vi "initialise.vi"(8 "error in (no error)":errorcluster, 11 "DL090202FPGAClock in":refnum<class "ClockDL090202FPGA.lvclass">) -> (0 "error out":errorcluster, 3 "DL090202FPGAClock out":refnum<class "ClockDL090202FPGA.lvclass">)   [LabVIEW 2010, in "ClockDL090202FPGA.lvclass"]
uses:
  ClockDL090202FPGA.lvclass
  GenericClock/GenericClock/GenericClock.lvclass
  ClockDL090202FPGA.lvclass/ClockDL090202FPGA.ctl
  FPGAWrapper/GenericFPGAWrapper/GenericFPGAWrapper/GenericFPGAWrapper.lvclass
  common/classes/ErrorController/ErrorController/class_data.vi
  common/classes/ErrorController/ErrorController/ErrorController.lvclass
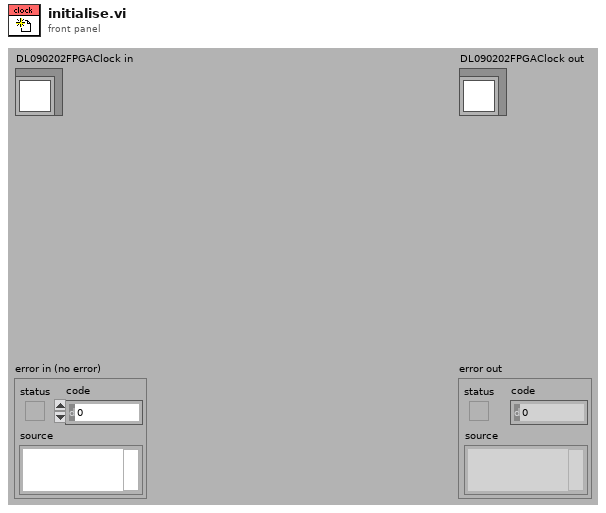
[diagram p1: front panel]
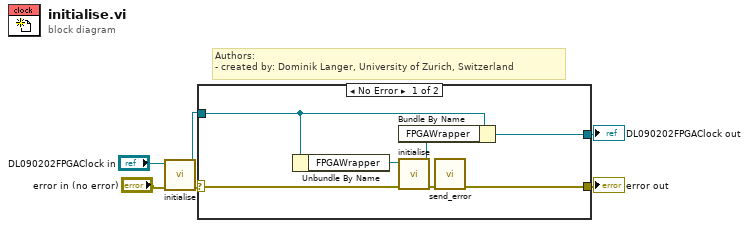
[diagram p0: block diagram]
diagram:
  # "Authors: \n- created by: Dominik Langer, University of Zurich, Switzerland"
  n1 = call-parent "initialise.vi"("error in (no error)"="error in (no error)", "GenericPlugin in"="DL090202FPGAClock in") -> ("error out"=w3:errorcluster, "GenericPlugin out"=w1:refnum<class "ClockDL090202FPGA.lvclass">)  [unwired: 8 out]
  n2 = case shown="No Error" w3 {
    selector: w3 -> [w11 w15]
    tunnel: [w7 w15] -> w6
    tunnel: [w12 w14] -> w5
    tunnel: w1 -> [w13 w14]
    frame No Error {
      n3 = Unbundle By Name(w13) -> ("FPGAWrapper"=w10:refnum<class "GenericFPGAWrapper.lvclass">)
      n4 = call-dynamic "initialise.vi"("error in (no error)"=w11, "GenericPlugin in"=w10) -> ("error out"=w8:errorcluster, "GenericPlugin out"=w9:refnum<class "GenericFPGAWrapper.lvclass">)  [unwired: 1 in, 7 out]
      n5 = Bundle By Name(cluster=w13, "FPGAWrapper"=w9) -> (w12:refnum<class "ClockDL090202FPGA.lvclass">)
      n6 = call "send_error.vi"("error in (no error)"=w8) -> ("error out"=w7:errorcluster)  [unwired: 10 in]
    }
    frame Error {
    }
  }
  "error out" <- w6
  "DL090202FPGAClock out" <- w5
